vi "Query Device.vi"(8 "error in":errorcluster, 11 "SR 3XX HVPS in":refnum<class "SR 3XX HVPS.lvclass">) -> (0 "error out":errorcluster, 2 "Dev":string, 3 "SR 3XX HVPS out":refnum<class "SR 3XX HVPS.lvclass">)   [LabVIEW 2014, in "SR 3XX HVPS.lvclass"]
doc: "The *IDN common query returns the PS300’s device configuration. This string is in the format: <B>StanfordResearchSystems,PS3XX,serial number, version number</B>, where XX is the particular model number, \"serial number\" is the serial number of the particular unit, and \"version number\" is the 3 digit firmware version number."
uses:
  SR 3XX HVPS.lvclass
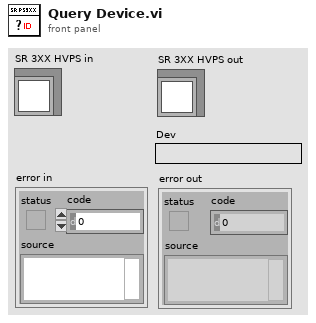
[diagram p1: front panel]
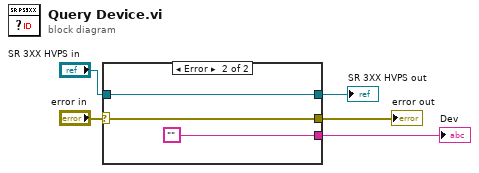
[diagram p0: block diagram]
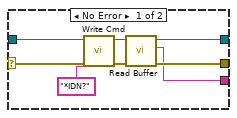
[diagram p2: hidden frame]
diagram:
  n1 = case shown="Error" "error in" {
    selector: "error in" -> [w9 w16]
    tunnel: [w7 w16] -> w4
    tunnel: [w8 w15] -> w2
    tunnel: "SR 3XX HVPS in" -> [w13 w15]
    tunnel: [w6 ""] -> w1
    frame No Error {
      n2 = call "Write Cmd.vi"("error in"=w9, "Cmd"="*IDN?", "SR 3XX HVPS in"=w13) -> ("error out"=w10:errorcluster, "SR 3XX HVPS out"=w11:refnum<class "SR 3XX HVPS.lvclass">)  [unwired: 7 in]
      n3 = call "Read Buffer.vi"("error in"=w10, "SR 3XX HVPS in"=w11) -> ("error out"=w7:errorcluster, "ReadData"=w6:string, "SR 3XX HVPS out"=w8:refnum<class "SR 3XX HVPS.lvclass">)  [unwired: 7 in]
    }
    frame Error {
    }
  }
  "error out" <- w4
  "SR 3XX HVPS out" <- w2
  "Dev" <- w1
